vi "Offset Locking- Main v0.1.vi"() -> ()   [LabVIEW 2017]
uses:
  <vilib>/Utility/error.llb/DialogType.ctl
  <vilib>/measure/mamon.llb/Waveform Peak Detection for 1 Chan.vi
  <vilib>/addons/control/pid/pid.llb/PID Advanced (DBL).vi
  <vilib>/measure/NI_MAPro.lvlib
  <vilib>/addons/control/pid/NI_PID_pid.lvlib
  <vilib>/Analysis/NI_AALBase.lvlib
panel:
  in  "# of Shots for Averaging":i32
  in  "Name Convention":string="FP 300MHz and WM 01"
  in  "Save Directory":path=path "C:/Users/LabUser/Google Drive/Measurements/11-2017"
  out "Three peaks?":bool
  out "Waveform Chart":dbl(graph)
  in  "PID Gains":T1={"proportional gain (Kc)"=1.0, "integral time (Ti, min)"=0.01, "derivative time (Td, min)"=0.0} {"derivative time (Td, min)" format="%.3f"; "integral time (Ti, min)" format="%.3f"; "proportional gain (Kc)" format="%.3f"}
  in  "Setpoint Range (GHz)":cluster{"setpoint high":dbl, "setpoint low":dbl}={"setpoint high"=100.0, "setpoint low"=0.0} {"setpoint high" format="%.3f"; "setpoint low" format="%.3f"}
  out "output":dbl format="%.2f"
  out "dt out (s)":dbl format="%.3f"
  in  "setpoint":dbl format="%.3f"
  out "GHz/sec":dbl
  out "dt":dbl format="%#_4g"
  out "Locations":dbl[](array[numeric]) format="%.2p"
  out "Amplitudes":dbl[](array[numeric]) format="%.2p"
  out "2nd Derivatives":dbl[](array[numeric]) format="%.2p"
  out "Waveform Graph":dynamicdata(graph)
  in  "Stop":bool
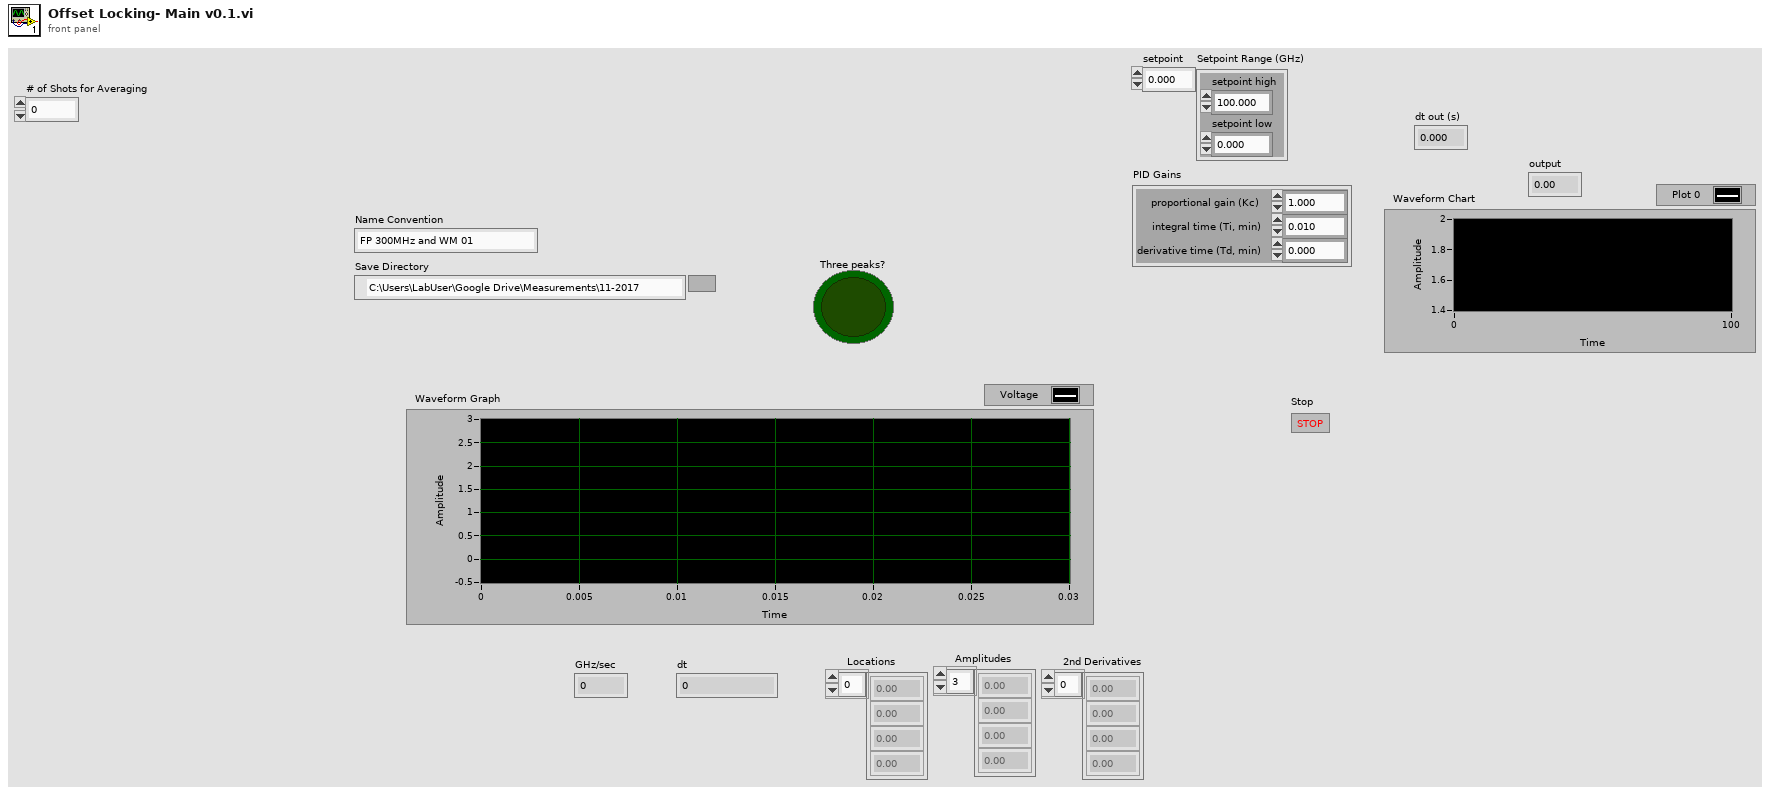
[diagram p1: front panel]
types:
  T1 = cluster{"proportional gain (Kc)":dbl, "integral time (Ti, min)":dbl, "derivative time (Td, min)":dbl}
  T2 = typedef "DialogType.ctl" = u16
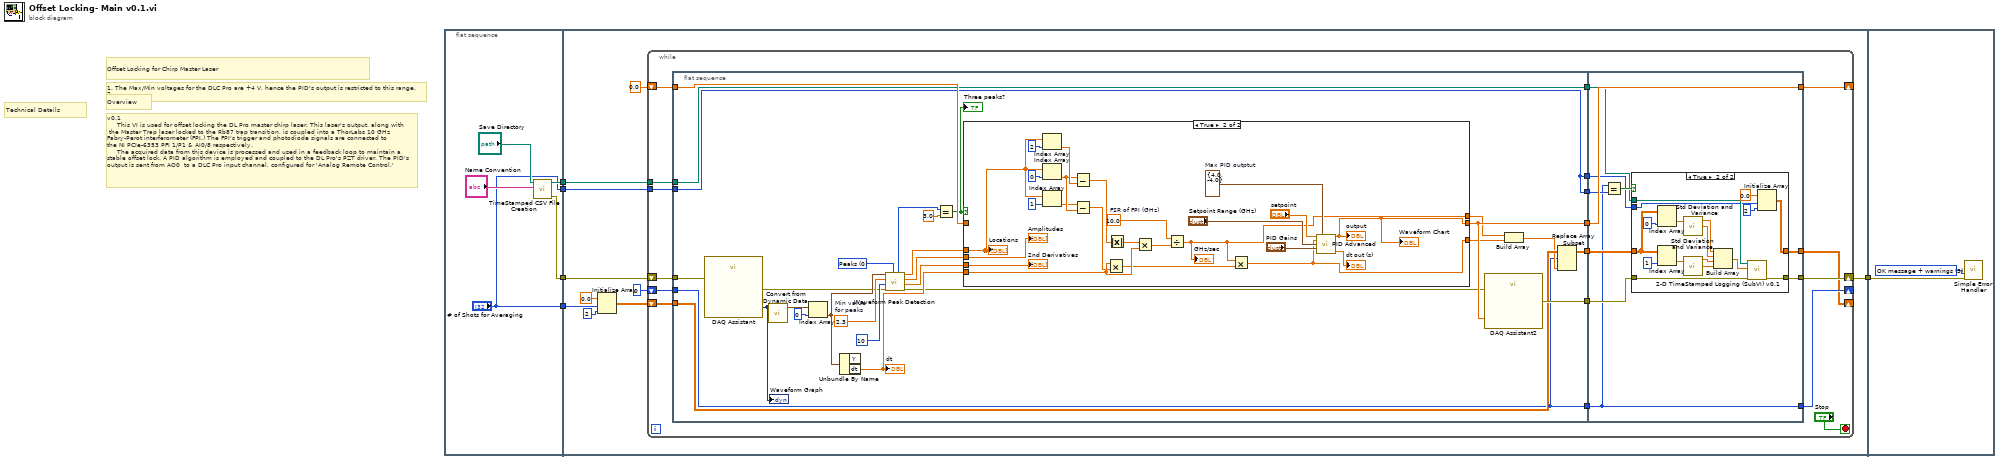
[diagram p0: block diagram]
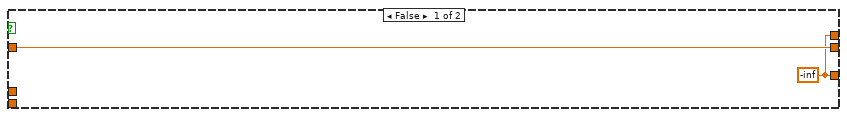
[diagram p2: hidden frame]
diagram:
  # "1. The Max/Min voltages for the DLC Pro are +4 V, hence the PID's output is restricted to this range.\n2."
  # "Technical Details"
  # "v0.1\n     This VI is used for offset locking the DL Pro master chirp laser. This laser's output, along with\n the Master Trap laser locked to the Rb87 trap transition, is coupled into a ThorLabs 10 GHz \nFabry-Perot interferometer (FPI.) The FPI's trigger and photodiode signals are connected to \nthe NI PCIe-6353 PFI 1/P1 & AI0/8 respectively. \n     The acquired data from this device is processed and used in a feedback loop to maintain a \nstable offset lock. A PID algorithm is employed and coupled to the DL Pro's PZT driver. The PID's\noutput is sent from AO0  to a DLC Pro input channel, configured for 'Analog Remote Control.'"
  # "Overview"
  # "Offset Locking for Chirp Master Laser"
  n1 = flat-sequence {
    tunnel: [w8] -> w5
    tunnel: ["# of Shots for Averaging"] -> w3
    tunnel: ["# of Shots for Averaging"] -> w2
    tunnel: [w6] -> w1
    tunnel: w5 -> [w19]
    tunnel: [w18] -> w4
    tunnel: w3 -> [w16]
    tunnel: w2 -> [w13]
    tunnel: w1 -> [w11]
    tunnel: w4 -> [w122]
    frame #0 {
      n2 = call "TimeStamped CSV File Creation.vi"("Name Convention"="Name Convention", "Save Directory"="Save Directory") -> ("error out"=w6:errorcluster, "path"=w8:path)  [unwired: 8 in]
    }
    frame #1 {
      n3 = Initialize Array(0.0 ("element"), w13, 2 ("dimension size")) -> (w15:dbl[][])
      n4 = while {
        shift-right: [w31] -> _
        shift-left: 0.0 -> [w37]
        shift-right: [w23] -> w18
        shift-left: w11 -> [w36]
        tunnel: w19 -> [w33]
        shift-right: [w22] -> _
        shift-left: 0 -> [w30]
        tunnel: w16 -> [w28]
        shift-right: [w21] -> _
        shift-left: w15 -> [w25]
        stop <- "Stop" stop-if-true
        n5 = flat-sequence {
          tunnel: w37 -> [w53]
          tunnel: w36 -> [w49]
          tunnel: [w51] -> w35
          tunnel: [w50] -> w34
          tunnel: w33 -> [w46]
          tunnel: [w46] -> w32
          tunnel: w30 -> [w39]
          tunnel: [w39] -> w29
          tunnel: w28 -> [w40]
          tunnel: [w40] -> w27
          tunnel: [w45] -> w26
          tunnel: w25 -> [w44]
          tunnel: [w40] -> w24
          tunnel: w35 -> [w102]
          tunnel: w34 -> [w95]
          tunnel: w32 -> [w96]
          tunnel: [w102] -> w31
          tunnel: w29 -> [w94]
          tunnel: w27 -> [w101]
          tunnel: w26 -> [w98]
          tunnel: w24 -> [w99]
          tunnel: [w97] -> w23
          tunnel: [w94] -> w22
          tunnel: [w93] -> w21
          frame #0 {
            w56 = u16 0 items=["Peaks", "Valleys"] ("peaks/valleys")
            w58 = 2.3  # Min value for peaks
            n6 = call "DAQ Assistant"("error in"=w49) -> ("data"=w64:dynamicdata, "error out"=w48:errorcluster)  [unwired: 16 in, 1 out]
            "Waveform Graph" <- w64
            n7 = call "Convert from Dynamic Data"("Dynamic Data Type"=w64) -> ("Array of Waveform"=w66:waveform(dbl)[])  [unwired: 3 in]
            n8 = Index Array(array=w66, index=0) -> (element=w61:waveform(dbl))
            n9 = Unbundle By Name(w61) -> ("dt"=w59:dbl)  [unwired: 1 out]
            "dt" <- w59
            n10 = call-poly <vilib>:"Waveform Peak Detection.vi"("peaks/valleys"=w56, "error in"=w48, "width"=10, "threshold"=w58, "Signal In"=w61) -> ("error out"=w47:errorcluster, "2nd Derivatives"=w62:dbl[], "Amplitudes"=w63:dbl[], "Locations"=w60:dbl[], "# found"=w54:i32)  [unwired: 2 in]
            n11 = Equal?(x=w54, y=3.0) -> (x = y?=w52:bool)
            "Three peaks?" <- w52
            n12 = case shown="True" w52 {
              tunnel: w63 -> [_ w90]
              tunnel: w62 -> [_ w89]
              tunnel: w60 -> [_ w82]
              tunnel: w59 -> [_ w78]
              tunnel: [w68 w71] -> w51
              tunnel: w53 -> [w68 _]
              tunnel: [w67 w70] -> w43
              tunnel: [w67 w69] -> w42
              frame False {
                w67 = -inf
              }
              frame True {
                w72 = cluster{"output high":dbl, "output low":dbl} {"output high"=4.0, "output low"=-4.0}  # Max PID outptut
                w87 = 10.0  # FSR of FPI (GHz)
                n13 = Index Array(array=w82, index=2) -> (element=w88:dbl)
                n14 = Index Array(array=w82, index=0 ("length")) -> (element=w81:dbl)
                n15 = Index Array(array=w82, index=1) -> (element=w80:dbl)
                n16 = Subtract(x=w81, y=w88) -> (x-y=w85:dbl)
                n17 = Subtract(x=w80, y=w81) -> (x-y=w79:dbl)
                n18 = Multiply(x=w78, y=w79) -> (x*y=w77:dbl)
                n19 = Absolute Value(x=w85) -> (abs(x)=w84:dbl)
                n20 = Multiply(x=w84, y=w78) -> (x*y=w86:dbl)
                n21 = Divide(x=w87, y=w86) -> (x/y=w70:dbl)
                "GHz/sec" <- w70
                n22 = Multiply(x=w70, y=w77) -> (x*y=w69:dbl)
                n23 = call-poly <vilib>:"PID Advanced.vi"("setpoint"="setpoint", "output range"=w72, "process variable"=w69, "setpoint range"="Setpoint Range (GHz)", "PID gains"="PID Gains") -> ("output"=w71:dbl, "dt out (s)"=→"dt out (s)":dbl)  [unwired: 9 in]
                "output" <- w71
                "Waveform Chart" <- w71
                "2nd Derivatives" <- w89
                "Amplitudes" <- w90
                "Locations" <- w82
              }
            }
            n24 = call "DAQ Assistant2"("data"=w51, "error in"=w47) -> ("error out"=w50:errorcluster)  [unwired: 16 in, 1 out]
            n25 = Build Array(w43, w42) -> (w41:dbl[])
            n26 = Replace Array Subset(array=w44, new element=w41, index (row)=w39) -> (w45:dbl[][])  [unwired: 1 in]
          }
          frame #1 {
            n27 = Equal?(x=w94, y=w101) -> (x = y?=w100:bool)
            n28 = case shown="True" w100 {
              tunnel: w99 -> [_ w106]
              tunnel: w98 -> [w103 w117]
              tunnel: [w104 w112] -> w97
              tunnel: w96 -> [_ w110]
              tunnel: w95 -> [w104 w109]
              tunnel: [w103 w105] -> w93
              frame False {
              }
              frame True {
                n29 = Index Array(array=w117, index (col)=0 ("disabled index (col)")) -> (element=w120:dbl[])  [unwired: 1 in]
                n30 = Index Array(array=w117, index (col)=1 ("disabled index (col)")) -> (element=w118:dbl[])  [unwired: 1 in]
                n31 = call <vilib>:"Std Deviation and Variance.vi"("X"=w120) -> ("mean"=w116:dbl, "standard deviation"=w115:dbl)  [unwired: 1 in, 1 out]
                n32 = call <vilib>:"Std Deviation and Variance.vi"("X"=w118) -> ("mean"=w114:dbl, "standard deviation"=w113:dbl)  [unwired: 1 in, 1 out]
                n33 = Build Array(w116, w115, w114, w113) -> (w111:dbl[])
                n34 = call "2-D TimeStamped Logging (SubVI) v0.1.vi"("error in (no error)"=w109, "array"=w111, "path"=w110) -> ("error out"=w112:errorcluster)  [unwired: 8 in]
                n35 = Initialize Array(0.0 ("element"), w106, 2 ("dimension size")) -> (w105:dbl[][])
              }
            }
          }
        }
      }
    }
    frame #2 {
      w123 = T2 3 items=["no dialog", "OK message", "continue or stop message", "OK message + warnings", "continue/stop + warnings"] ("type of dialog (OK msg:1)")
      n36 = call <vilib>:"Simple Error Handler.vi"("type of dialog (OK msg:1)"=w123, "error in (no error)"=w122) -> ()  [unwired: 3 in, 5 out]
    }
  }
